vi "OAT Output Trigger Event (cluster of x0, dx, array).vi"(0 "signal in":cluster{"x0":dbl, "dx":dbl, "array":dbl[]}={"x0"=0.0, "dx"=1.0, "array"=[]} {"array" format="%.2f"; "dx" format="%.2p"; "x0" format="%.2p"}, 1 "trigger on":T1(ring), 2 "reset? (F)":bool, 5 "upper setpoint":dbl=inf, 7 "lower setpoint":dbl=-inf, 9 "hysteresis":dbl format="%.2p", 11 "error in (no error)":errorcluster) -> (4 "trigger detected?":bool, 15 "error out":errorcluster)   [LabVIEW 2017, in "SoundVib_OAUtility.lvlib"]
doc: "Detects the first level-crossing condition. The <B>upper setpoint</B> and <B>lower setpoint</B> of the threshold and the <B>hysteresis</B> specify the trigger conditions. Wire data to the <B>signal in</B> input to determine the polymorphic instance to use or manually select the instance."
uses:
  <vilib>/addons/Sound and Vibration/Order Analysis/Utility/SoundVib_OAUtility.lvlib
  <vilib>/measure/mamon.llb/Trigger Detection for 1 Channel.vi
  <vilib>/measure/NI_MAPro.lvlib
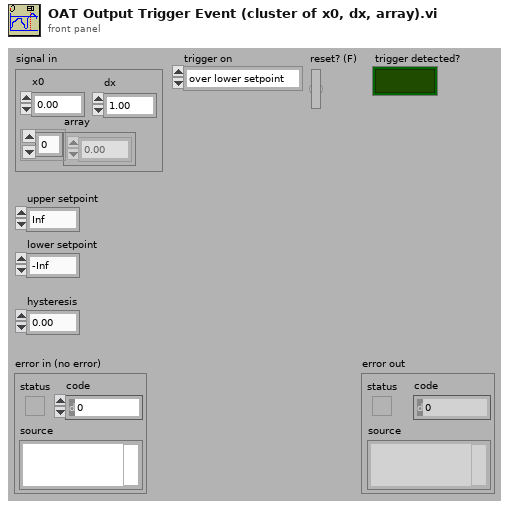
[diagram p1: front panel]
types:
  T1 = enum16{"over lower setpoint", "under upper setpoint", "both"}
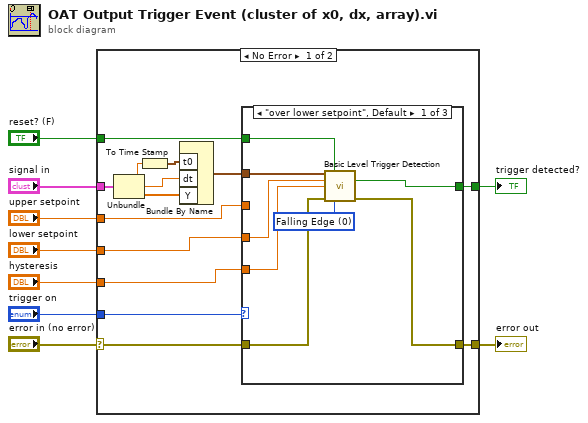
[diagram p0: block diagram]
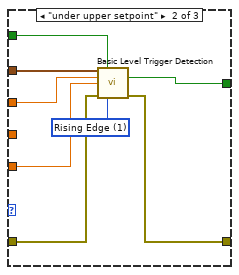
[diagram p2: hidden frame]
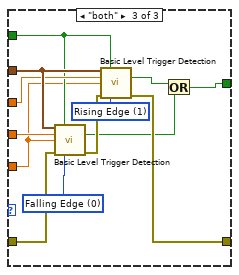
[diagram p3: hidden frame]
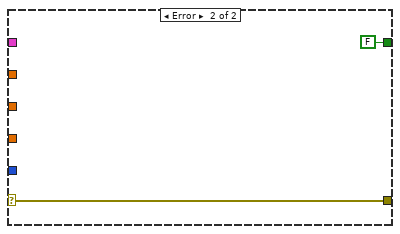
[diagram p4: hidden frame]
diagram:
  n1 = case shown="No Error" "error in (no error)" {
    selector: "error in (no error)" -> [w12 w54]
    tunnel: [w11 w54] -> w8
    tunnel: "signal in" -> [w23 _]
    tunnel: "reset? (F)" -> [w17 _]
    tunnel: "upper setpoint" -> [w16 _]
    tunnel: "lower setpoint" -> [w15 _]
    tunnel: "hysteresis" -> [w14 _]
    tunnel: "trigger on" -> [w13 _]
    tunnel: [w10 FALSE ("trigger detected?")] -> w1
    frame No Error {
      n2 = Unbundle(w23) -> ("x0"=w20:dbl, "dx"=w21:dbl, "array"=w22:dbl[])
      n3 = To Time Stamp(1:w20) -> (0:w19:timestamp)
      n4 = Bundle By Name("t0"=w19, "dt"=w21, "Y"=w22) -> (w18:waveform(dbl))  [unwired: 1 in]
      n5 = case shown="\"over lower setpoint\", Default" w13 {
        tunnel: w18 -> [w31 w39 w52]
        tunnel: w17 -> [w30 w38 w41]
        tunnel: w15 -> [w28 _ w50]
        tunnel: w12 -> [w27 w36 w47]
        tunnel: [w26 w33 w45] -> w11
        tunnel: [w25 w34 w42] -> w10
        tunnel: w16 -> [_ w37 w51]
        tunnel: w14 -> [w24 w32 w40]
        frame "over lower setpoint", Default {
          w29 = u16 0 items=["Falling Edge", "Rising Edge"] ("slope")
          n6 = call-poly <vilib>:"Basic Level Trigger Detection.vi"("signal in"=w31, "reset"=w30, "level"=w28, "hysteresis"=w24, "error in (no error)"=w27, "trigger slope"=w29) -> ("trigger detected?"=w25:bool, "error out"=w26:errorcluster)  [unwired: 7 in, 1 out]
        }
        frame "under upper setpoint" {
          w35 = u16 1 items=["Falling Edge", "Rising Edge"] ("slope")
          n7 = call-poly <vilib>:"Basic Level Trigger Detection.vi"("signal in"=w39, "reset"=w38, "level"=w37, "hysteresis"=w32, "error in (no error)"=w36, "trigger slope"=w35) -> ("trigger detected?"=w34:bool, "error out"=w33:errorcluster)  [unwired: 7 in, 1 out]
        }
        frame "both" {
          w48 = u16 0 items=["Falling Edge", "Rising Edge"] ("slope")
          w49 = u16 1 items=["Falling Edge", "Rising Edge"] ("slope")
          n8 = call-poly <vilib>:"Basic Level Trigger Detection.vi"("signal in"=w52, "reset"=w41, "level"=w50, "hysteresis"=w40, "error in (no error)"=w47, "trigger slope"=w48) -> ("trigger detected?"=w43:bool, "error out"=w46:errorcluster)  [unwired: 7 in, 1 out]
          n9 = call-poly <vilib>:"Basic Level Trigger Detection.vi"("signal in"=w52, "reset"=w41, "level"=w51, "hysteresis"=w40, "error in (no error)"=w46, "trigger slope"=w49) -> ("trigger detected?"=w44:bool, "error out"=w45:errorcluster)  [unwired: 7 in, 1 out]
          n10 = Or(x=w44, y=w43) -> (x .or. y?=w42:bool)
        }
      }
    }
    frame Error {
    }
  }
  "error out" <- w8
  "trigger detected?" <- w1
